vi "Check if Path Is Test.vi"(9 "Path":path) -> (1 "IsTest?":bool)   [LabVIEW 2011, in "VITesterUtilities.lvlib"]
uses:
  Libraries/VITesterUtilities.lvlib
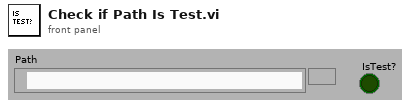
[diagram p1: front panel]
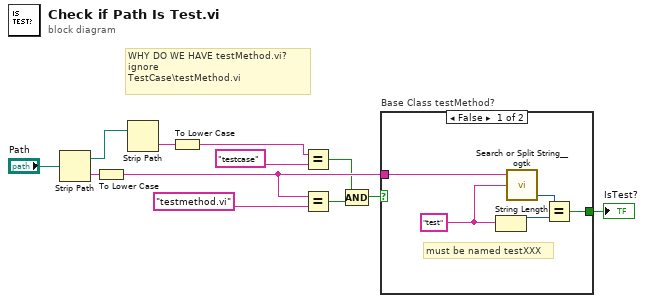
[diagram p0: block diagram]
diagram:
  # "WHY DO WE HAVE testMethod.vi?\nignore\nTestCase\\testMethod.vi"
  n1 = Strip Path(path="Path") -> (stripped path=w9:path, name=w12:string)
  n2 = To Lower Case(string=w12) -> (all lower case string=w5:string)
  n3 = Strip Path(path=w9) -> (name=w8:string)  [unwired: 1 out]
  n4 = To Lower Case(string=w8) -> (all lower case string=w7:string)
  n5 = Equal?(x=w7, y="testcase" ("search string/char (-)")) -> (x = y?=w2:bool)
  n6 = Equal?(x=w5, y="testmethod.vi" ("search string/char (-)")) -> (x = y?=w3:bool)
  n7 = Compound Arithmetic op=AND(w2, w3) -> (w1:bool)
  n8 = case "Base Class testMethod?" shown="False" w1 {
    tunnel: [w17 _] -> w11
    tunnel: w5 -> [w13 _]
    frame False {
      w15 = "test" ("search string/char (-)")
      # "must be named testXXX"
      n9 = String Length(string=w15) -> (length=w16:i32)
      n10 = call <userlib>:"Search or Split String__ogtk.vi"("search string/char (-)"=w15, "string"=w13) -> ("offset after match"=w14:i32)  [unwired: 1 in, 2 out]
      n11 = Equal?(x=w14, y=w16) -> (x = y?=w17:bool)
    }
    frame True {
      # "ignore base class Test method."
    }
  }
  "IsTest?" <- w11
